vi "FROG.vi"(8 "wl_min_max":dbl[](array[numeric]), 9 "data":dbl[][](array[numeric]), 10 "wl":dbl[](array[numeric]), 11 "time":dbl[](array[numeric])) -> ()   [LabVIEW 2019]
panel:
  out "XY Graph":cluster{dbl[], "time":dbl[]}(graph)
  out "XY Graph 2":cluster{dbl[], dbl[]}(graph)
  out "Intensity Graph":dbl[][](graph)
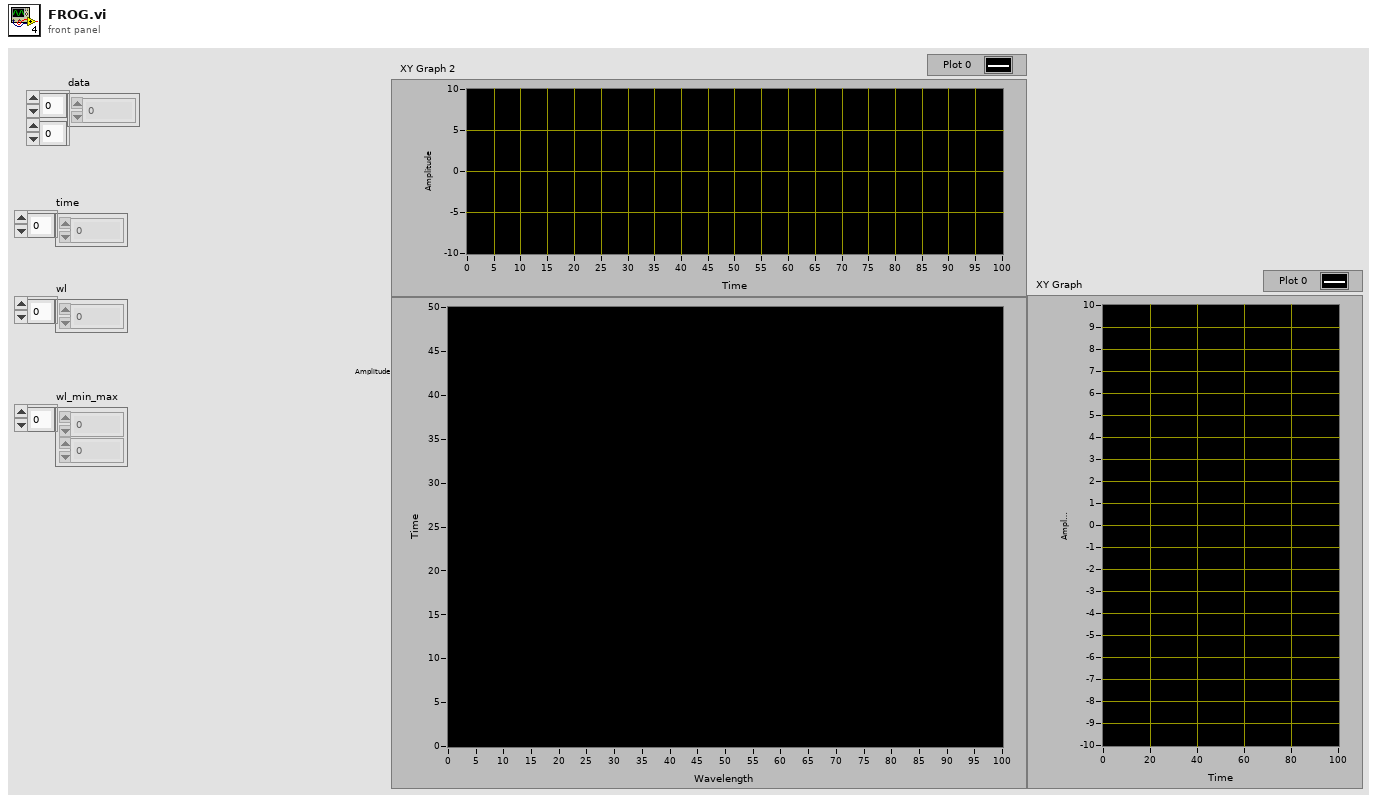
[diagram p1: front panel]
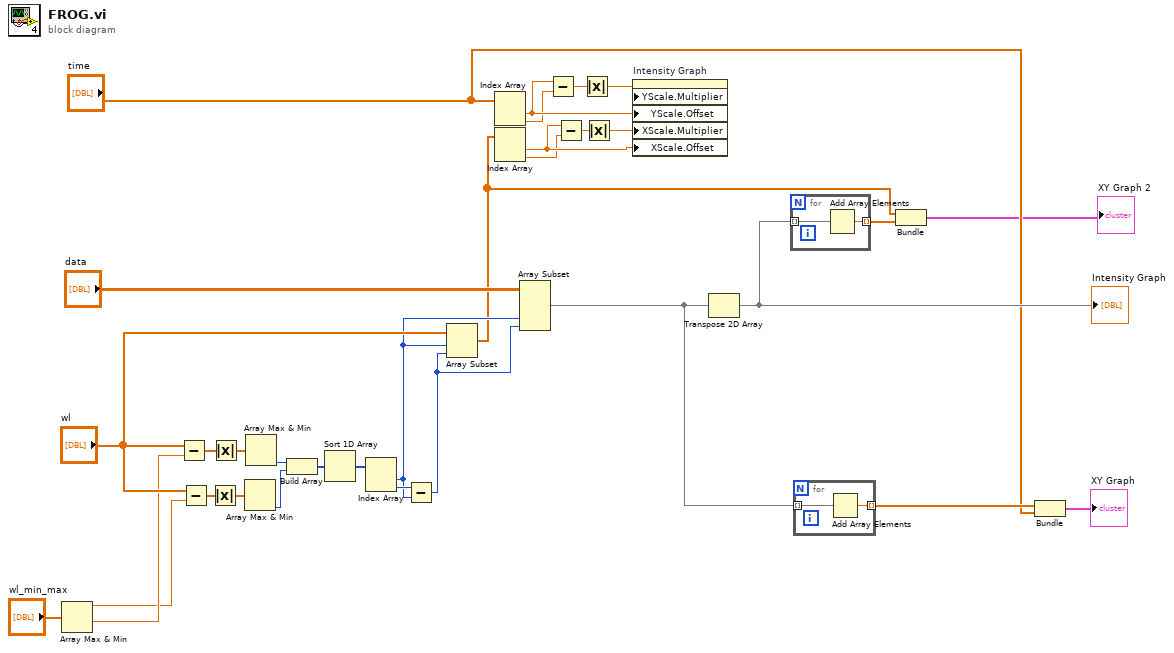
[diagram p0: block diagram]
diagram:
  n1 = Array Max & Min(array="wl_min_max") -> (max value=w1:dbl, min value=w2:dbl)  [unwired: 2 out]
  n2 = Subtract(x="wl", y=w2) -> (x-y=w32:dbl[])
  n3 = Subtract(x="wl", y=w1) -> (x-y=w30:dbl[])
  n4 = Absolute Value(x=w30) -> (abs(x)=w29:dbl[])
  n5 = Absolute Value(x=w32) -> (abs(x)=w31:dbl[])
  n6 = Array Max & Min(array=w29) -> (min index (indices)=w26:i32)  [unwired: 3 out]
  n7 = Array Max & Min(array=w31) -> (min index (indices)=w27:i32)  [unwired: 3 out]
  n8 = Build Array(w27, w26) -> (w25:i32[])
  n9 = Sort 1D Array(array=w25) -> (sorted array=w24:i32[])
  n10 = Index Array(array=w24) -> (element #1=w17:i32, element #2=w23:i32)  [unwired: 2 in]
  n11 = Subtract(x=w23, y=w17) -> (x-y=w16:i32)
  n12 = Array Subset(array="wl", index=w17, length=w16) -> (w5:dbl[])
  n13 = Index Array(array="time") -> (element #1=w22:dbl, element #2=w21:dbl)  [unwired: 2 in]
  n14 = Index Array(array=w5) -> (element #1=w15:dbl, element #2=w14:dbl)  [unwired: 2 in]
  n15 = Array Subset(array="data", index (col)=w17, length (col)=w16) -> (w10:dbl[][])  [unwired: 2 in]
  n16 = Subtract(x=w22, y=w21) -> (x-y=w20:dbl)
  n17 = Subtract(x=w15, y=w14) -> (x-y=w13:dbl)
  n18 = Absolute Value(x=w20) -> (abs(x)=w19:dbl)
  n19 = Absolute Value(x=w13) -> (abs(x)=w12:dbl)
  n20 = property on="Intensity Graph" class="IntGraph (strict)"("YScale.Multiplier"=w19, "YScale.Offset"=w22, "XScale.Multiplier"=w12, "XScale.Offset"=w15) -> ()  [unwired: 2 in, 2 out]
  n21 = Transpose 2D Array(2D array=w10) -> (transposed array=w11:dbl[][])
  "Intensity Graph" <- w11
  n22 = for {
    tunnel: w11 -> [w34] mode=indexing
    tunnel: [w33] -> w6 mode=indexing
    n23 = Add Array Elements(numeric array=w34) -> (sum=w33:dbl)
  }
  n24 = for {
    tunnel: w10 -> [w36] mode=indexing
    tunnel: [w35] -> w9 mode=indexing
    n25 = Add Array Elements(numeric array=w36) -> (sum=w35:dbl)
  }
  n26 = Bundle(w5, w6) -> (→"XY Graph 2":cluster{dbl[], dbl[]})  [unwired: 1 in]
  n27 = Bundle(w9, "time"="time") -> (→"XY Graph":cluster{dbl[], "time":dbl[]})  [unwired: 1 in]
